vi "GUI.Close.vi"(11 "State Variables in":T1) -> ()   [LabVIEW 2025, in "XNET Bus Monitor Client.lvlib"]
uses:
  XNET Bus Monitor Client.lvlib
  Types/GUI.StateVariables.ctl
  Types/GUI.Controls.Refs.ctl
  bus_monitor_client/RPC Messages/ni_bus_monitor_api_DirectionFilter.ctl
  bus_monitor_client/RPC Messages/ni_bus_monitor_api_FrameFilter.ctl
  Types/StreamEngine.QueueRefs.ctl
  Types/StreamEngine.CmdQueueData.ctl
  Types/StreamEngine.CmdQueueData.Cmd.ctl
  Types/SubProcessEngine.QueueRefs.ctl
  Types/SubProcessEngine.CmdQueueData.ctl
  Types/SubProcessEngine.CmdQueueData.Cmd.ctl
  Types/gRPC.ConnectionInfo.ctl
  <vilib>/gRPC/LabVIEW gRPC Library/Shared/grpcId.ctl
  bus_monitor_client/RPC Messages/ni_bus_monitor_api_Session.ctl
  bus_monitor_client/bus_monitor_client.lvlib
  <vilib>/gRPC/LabVIEW gRPC Library/grpc-lvsupport-release.lvlib
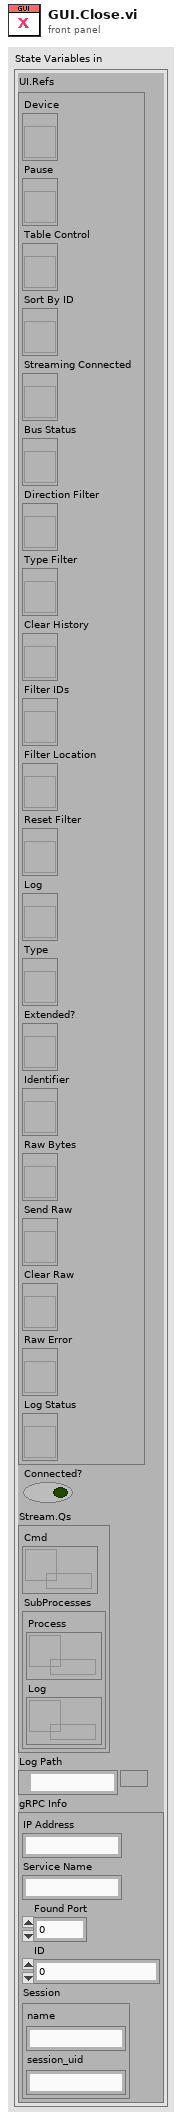
[diagram p1: front panel]
types:
  T1 = typedef "XNET Bus Monitor Client.lvlib/GUI.StateVariables.ctl" = cluster{"UI.Refs":T2, "Connected?":bool, "Stream.Qs":T3, "Log Path":path, "gRPC Info":T5}
  T2 = typedef "XNET Bus Monitor Client.lvlib/GUI.Controls.Refs.ctl" = cluster{"Device":refnum<vi>, "Pause":refnum<vi>, "Table Control":refnum<vi>, "Sort By ID":refnum<vi>, "Streaming Connected":refnum<vi>, "Bus Status":refnum<vi>, "Direction Filter":refnum<vi>, "Type Filter":refnum<vi>, "Clear History":refnum<vi>, "Filter IDs":refnum<vi>, "Filter Location":refnum<vi>, "Reset Filter":refnum<vi>, "Log":refnum<vi>, "Type":refnum<vi>, "Extended?":refnum<vi>, "Identifier":refnum<vi>, "Raw Bytes":refnum<vi>, "Send Raw":refnum<vi>, "Clear Raw":refnum<vi>, "Raw Error":refnum<vi>, "Log Status":refnum<vi>}
  T3 = typedef "XNET Bus Monitor Client.lvlib/StreamEngine.QueueRefs.ctl" = cluster{"Cmd":refnum<queue>, "SubProcesses":T4}
  T4 = typedef "XNET Bus Monitor Client.lvlib/SubProcessEngine.QueueRefs.ctl" = cluster{"Process":refnum<queue>, "Log":refnum<queue>}
  T5 = typedef "XNET Bus Monitor Client.lvlib/gRPC.ConnectionInfo.ctl" = cluster{"IP Address":string, "Service Name":string, "Found Port":u64, "ID":T6, "Session":T7}
  T6 = typedef "grpc-lvsupport-release.lvlib/grpcId.ctl" = u64
  T7 = typedef "bus_monitor_client.lvlib/ni_bus_monitor_api_Session.ctl" = cluster{"name":string, "session_uid":string}
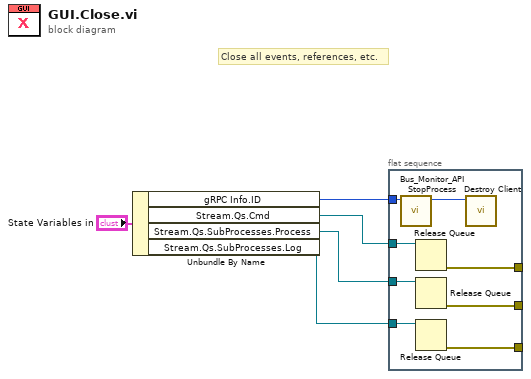
[diagram p0: block diagram]
diagram:
  # "Close all events, references, etc."
  n1 = Unbundle By Name("State Variables in") -> ("gRPC Info.ID"=w4:T6, "Stream.Qs.Cmd"=w3:refnum<queue>, "Stream.Qs.SubProcesses.Process"=w2:refnum<queue>, "Stream.Qs.SubProcesses.Log"=w1:refnum<queue>)
  n2 = flat-sequence {
    tunnel: w4 -> [w13]
    tunnel: w3 -> [w11]
    tunnel: w2 -> [w10]
    tunnel: w1 -> [w9]
    tunnel: [w8] -> _
    tunnel: [w7] -> _
    tunnel: [w6] -> _
    frame #0 {
      n3 = call "Bus_Monitor_API StopProcess.vi"("gRPC ID"=w13) -> ("gRPC ID out"=w12:T6)  [unwired: 8 in, 2 out]
      n4 = Release Queue(queue=w11) -> (error out=w8:errorcluster)  [unwired: 2 in, 2 out]
      n5 = Release Queue(queue=w10) -> (error out=w7:errorcluster)  [unwired: 2 in, 2 out]
      n6 = Release Queue(queue=w9) -> (error out=w6:errorcluster)  [unwired: 2 in, 2 out]
      n7 = call "Destroy Client.vi"("gRPC ID"=w12) -> ()  [unwired: 10 in, 1 out]
    }
  }
